vi "Popup window-Cursor value entry management.vi"(4 "Rightcursor position":dbl, 6 "Left cursor position":dbl, 8 "error in":errorcluster, 9 "Right control ref":refnum<vi>, 10 "Left control ref":refnum<vi>, 11 "Timeline Ref in":T1) -> (0 "error out":errorcluster, 3 "XYGraph out":T1)   [LabVIEW 2017, in "XGrapher.xctl"]
uses:
  XGrapher.xctl
  Typedefs/Xctrl-Timeline graph ref.ctl
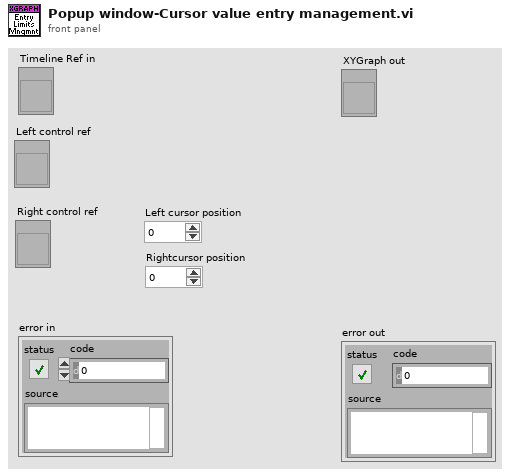
[diagram p1: front panel]
types:
  T1 = typedef "XGrapher.xctl/Xctrl-Timeline graph ref.ctl" = refnum<vi>
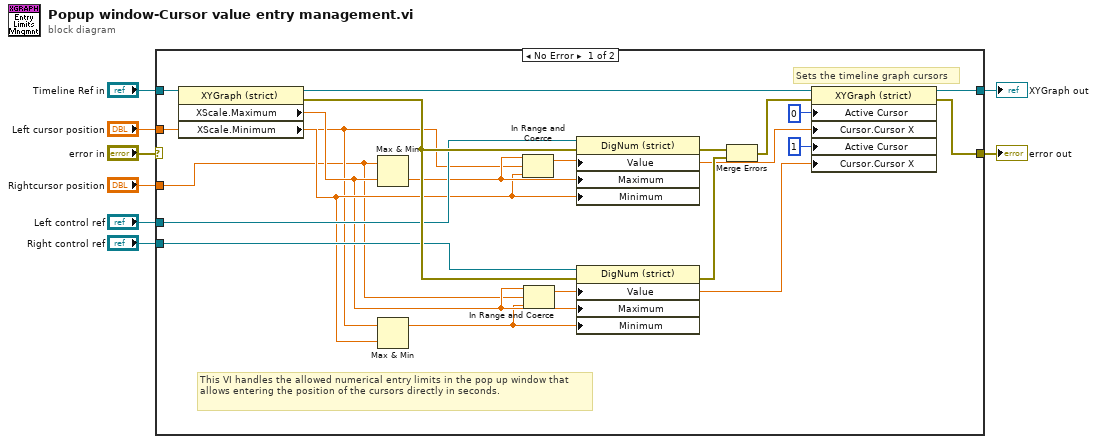
[diagram p0: block diagram]
diagram:
  n1 = case shown="No Error" "error in" {
    selector: "error in" -> [_ w30]
    tunnel: [w12 w30] -> w8
    tunnel: "Timeline Ref in" -> [w25 w29]
    tunnel: [w13 w29] -> w6
    tunnel: "Left control ref" -> [w24 _]
    tunnel: "Right control ref" -> [w23 _]
    tunnel: "Left cursor position" -> [w18 _]
    tunnel: "Rightcursor position" -> [w17 _]
    frame No Error {
      # "Sets the timeline graph cursors"
      # "This VI handles the allowed numerical entry limits in the pop up window that allows entering the position of the cursors directly in seconds."
      n2 = property on="Property Node" class="XYGraph (strict)"(reference=w25) -> (reference out=w14:T1, error out=w26:errorcluster, "XScale.Maximum"=w20:dbl, "XScale.Minimum"=w21:dbl)  [unwired: 1 in]
      n3 = Max & Min(x=w17, y=w20) -> (min(x,y)=w22:dbl)  [unwired: 1 out]
      n4 = Max & Min(x=w18, y=w21) -> (max(x,y)=w19:dbl)  [unwired: 1 out]
      n5 = In Range and Coerce(upper limit=w22, x=w18, lower limit=w21) -> (coerced(x)=w10:dbl)  [unwired: 1 out]
      n6 = In Range and Coerce(upper limit=w20, x=w17, lower limit=w19) -> (coerced(x)=w9:dbl)  [unwired: 1 out]
      n7 = property on="Property Node" class="DigNum (strict)"(reference=w24, error in=w26, "Value"=w10, "Maximum"=w22, "Minimum"=w21) -> (error out=w28:errorcluster)  [unwired: 1 out]
      n8 = property on="Property Node" class="DigNum (strict)"(reference=w23, error in=w26, "Value"=w9, "Maximum"=w20, "Minimum"=w19) -> (error out=w27:errorcluster)  [unwired: 1 out]
      n9 = Merge Errors(w28, w27) -> (w11:errorcluster)
      n10 = property on="Property Node" class="XYGraph (strict)"(reference=w14, error in=w11, "Active Cursor"=u32 0, "Cursor.Cursor X"=w10, "Active Cursor"=u32 1, "Cursor.Cursor X"=w9) -> (reference out=w13:T1, error out=w12:errorcluster)
    }
    frame Error {
    }
  }
  "error out" <- w8
  "XYGraph out" <- w6
